vi "Update DAC to evap.vi"(9 "Control array":T1(array[cluster]), 10 "Evasp calc'd time":dbl, 11 "In Array":T2(array[cluster])) -> (3 "Out Array":T2(array[cluster]))   [LabVIEW 2017]
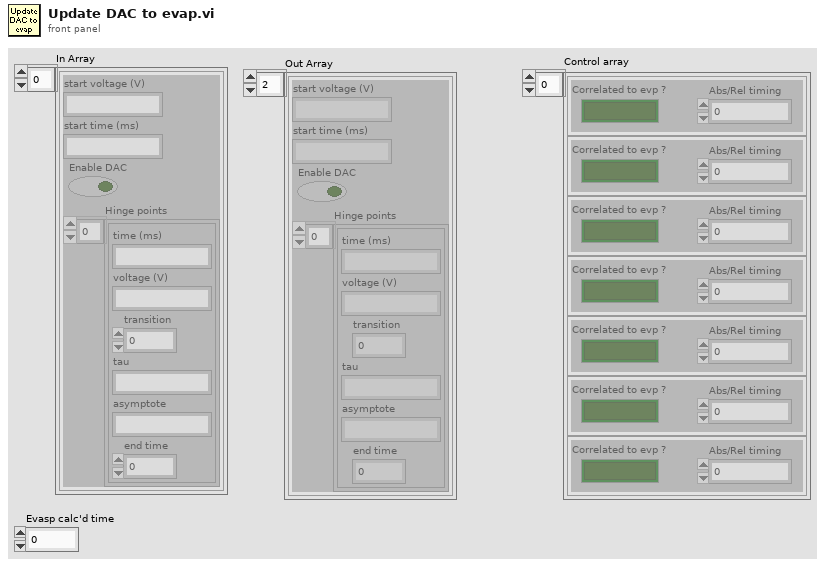
[diagram p1: front panel]
types:
  T1 = cluster{"Correlated to evp ?":bool, "Abs/Rel timing":dbl}[]
  T2 = cluster{"start voltage (V)":string, "start time (ms)":string, "Enable DAC":bool, "Hinge points":cluster{"time (ms)":string, "voltage (V)":string, "transition":u16, "tau":string, "asymptote":string, "end time":dbl}[]}[]
  T3 = cluster{"time (ms)":string, "voltage (V)":string, "transition":u16, "tau":string, "asymptote":string, "end time":dbl}[]
  T4 = cluster{"time (ms)":string, "voltage (V)":string, "transition":u16, "tau":string, "asymptote":string, "end time":dbl}
  T5 = cluster{"start voltage (V)":string, "start time (ms)":string, "Enable DAC":bool, "Hinge points":cluster{"time (ms)":string, "voltage (V)":string, "transition":u16, "tau":string, "asymptote":string, "end time":dbl}[]}
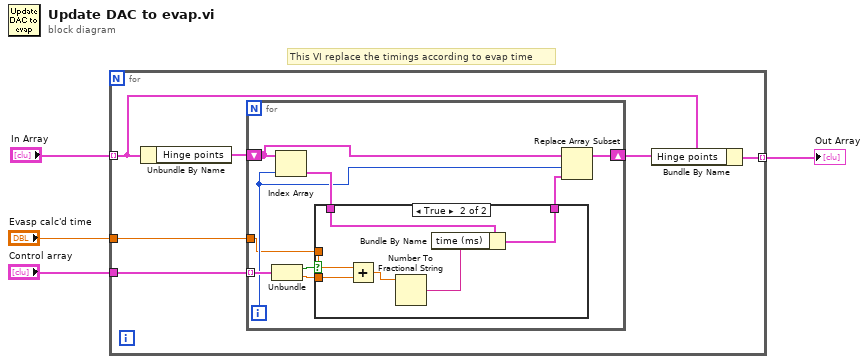
[diagram p0: block diagram]
diagram:
  # "This VI replace the timings according to evap time"
  n1 = for {
    tunnel: "Control array" -> [w10]
    tunnel: "In Array" -> [w7] mode=indexing
    tunnel: "Evasp calc'd time" -> [w9]
    tunnel: [w5] -> w1 mode=indexing
    n2 = Unbundle By Name(w7) -> ("Hinge points"=w8:T3)
    n3 = for {
      tunnel: w10 -> [w19] mode=indexing
      shift-right: [w16] -> w6
      shift-left: w8 -> [w15]
      tunnel: w9 -> [w12]
      i -> [w14]
      n4 = Unbundle(w19) -> ("Correlated to evp ?"=w18:bool, "Abs/Rel timing"=w11:dbl)
      n5 = Index Array(array=w15, index=w14) -> (element=w17:T4)
      n6 = case shown="True" w18 {
        tunnel: w17 -> [w20 w23]
        tunnel: [w20 w21] -> w13
        tunnel: w12 -> [_ w26]
        tunnel: w11 -> [_ w25]
        frame False {
        }
        frame True {
          n7 = Add(x=w26, y=w25) -> (x+y=w24:dbl)
          n8 = Number To Fractional String(number=w24) -> (F-format string=w22:string)  [unwired: 3 in]
          n9 = Bundle By Name(cluster=w23, "time (ms)"=w22) -> (w21:T4)
        }
      }
      n10 = Replace Array Subset(array=w15, new element=w13, index=w14) -> (w16:T3)
    }
    n11 = Bundle By Name(cluster=w7, "Hinge points"=w6) -> (w5:T5)
  }
  "Out Array" <- w1
